vi "Image default.vi"(7 "Label Text":string[](array[string]), 8 "error in (no error)":errorcluster, 11 "Ctl Refnum in":refnum<vi>) -> (0 "error out":errorcluster, 3 "Ctl Refnum out":refnum<vi>)   [LabVIEW 2017, in "Toolbox.lvlib"]
uses:
  Toolbox.lvlib
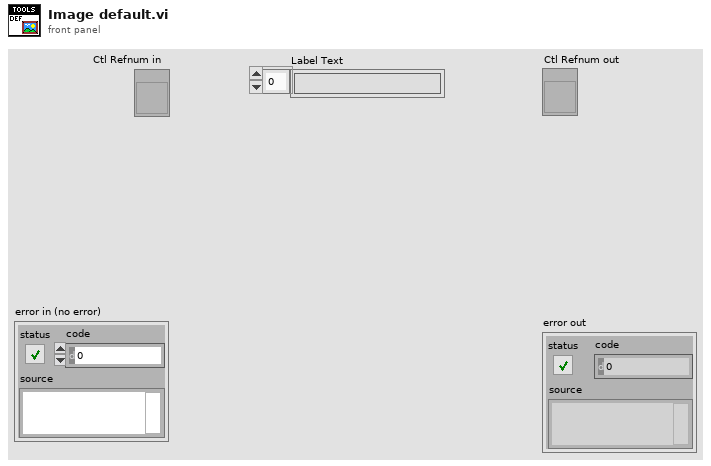
[diagram p1: front panel]
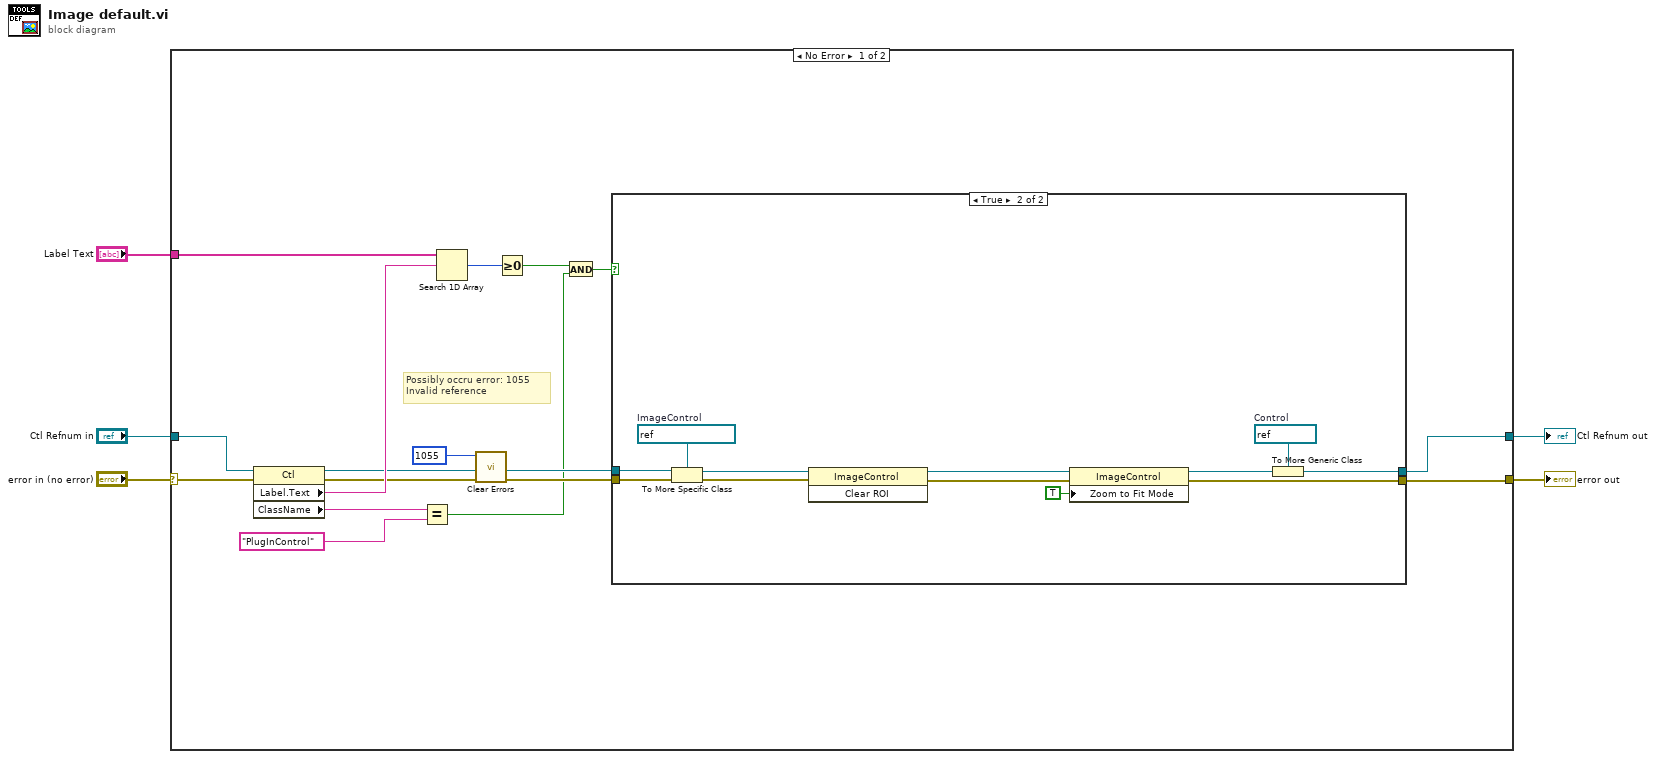
[diagram p0: block diagram]
diagram:
  n1 = case shown="No Error" "error in (no error)" {
    selector: "error in (no error)" -> [w21 w37]
    tunnel: [w14 w37] -> w4
    tunnel: "Ctl Refnum in" -> [w20 w36]
    tunnel: "Label Text" -> [w19 _]
    tunnel: [w11 w36] -> w1
    frame No Error {
      # "Possibly occru error: 1055\nInvalid reference"
      n2 = property class="Ctl"(reference=w20, error in=w21) -> (reference out=w16:refnum<vi>, error out=w17:errorcluster, "Label.Text"=w18:string, "ClassName"=w10:string)
      n3 = Equal?(x=w10, y="PlugInControl") -> (x = y?=w6:bool)
      n4 = Search 1D Array(1D array=w19, element=w18) -> (index of element=w15:i32)  [unwired: 1 in]
      n5 = call <vilib>:"Clear Errors.vi"("error in (no error)"=w17, "specific error code to clear (0: all)"=1055) -> ("error out"=w13:errorcluster)  [unwired: 4 in, 1 out]
      n6 = Greater Or Equal To 0?(x=w15) -> (x >= 0?=w7:bool)
      n7 = And(x=w7, y=w6) -> (x .and. y?=w8:bool)
      n8 = case shown="True" w8 {
        tunnel: w13 -> [w23 w35]
        tunnel: w16 -> [w22 w33]
        tunnel: [w23 w27] -> w14
        tunnel: [w22 w30] -> w11
        frame False {
        }
        frame True {
          w29 = refnum<vi> refnum  # Control
          w31 = refnum<vi> refnum  # ImageControl
          n9 = To More Specific Class(target class=w31, reference=w33, error in=w35) -> (specific class reference=w32:refnum<vi>, error out=w34:errorcluster)
          n10 = invoke class="ImageControl" method="Clear ROI"(reference=w32, error in=w34) -> (reference out=w26:refnum<vi>, error out=w28:errorcluster)  [unwired: 1 in, 1 out]
          n11 = property class="ImageControl"(reference=w26, error in=w28, "Zoom to Fit Mode"=TRUE) -> (reference out=w25:refnum<vi>, error out=w27:errorcluster)
          n12 = To More Generic Class(target class=w29, reference=w25) -> (generic class reference=w30:refnum<vi>)
        }
      }
    }
    frame Error {
    }
  }
  "error out" <- w4
  "Ctl Refnum out" <- w1
